vi "Simulated HW Control Panel (Tank).vi"() -> ()   [LabVIEW 2017, in "Simulated HW.lvclass"]
uses:
  Simulated HW.lvclass
panel:
  in  "Exhaust Valve State":dbl(slide) scale=0.0..5.0
  in  "Flow Valve State":dbl(slide) scale=0.0..5.0
  in  "Tank Pressure":dbl(slide) scale=0.0..200.0
  in  "Bottom":dbl(slide) scale=0.0..200.0
  in  "Middle":dbl(slide) scale=0.0..200.0
  in  "Top":dbl(slide) scale=0.0..200.0
  # "Tank Thermocouples"
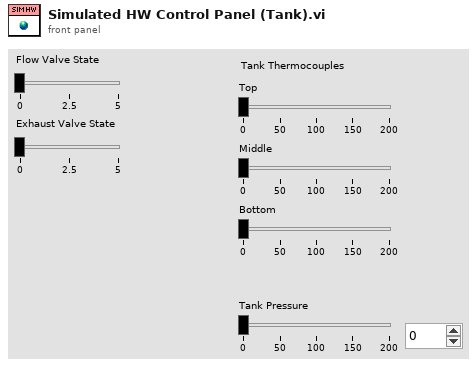
[diagram p1: front panel]
diagram:
